vi "Error Query.vi"(8 "error in (no error)":errorcluster, 11 "VISA resource name":refnum<visa-resource-name>) -> (0 "error out":errorcluster, 1 "Error Message":string, 2 "Error":i32, 3 "VISA resource name out":refnum<visa-resource-name>)   [LabVIEW 2011, in "Agilent 4194.lvlib"]
doc: "This function reads an error code from the instrument's error queue.\n\nNotes:\n\n(1) For list of error messages see also operation manual.\n\n(2)This instrument does not return an error message string."
uses:
  <instrlib>/Agilent 4194/Agilent 4194.lvlib
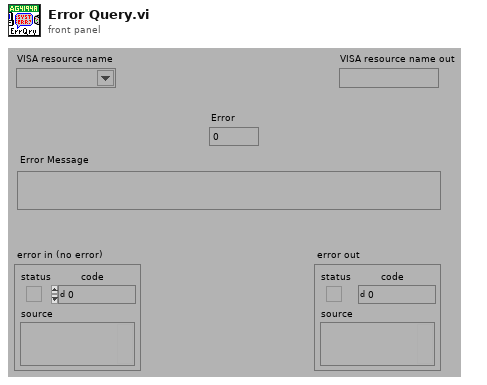
[diagram p1: front panel]
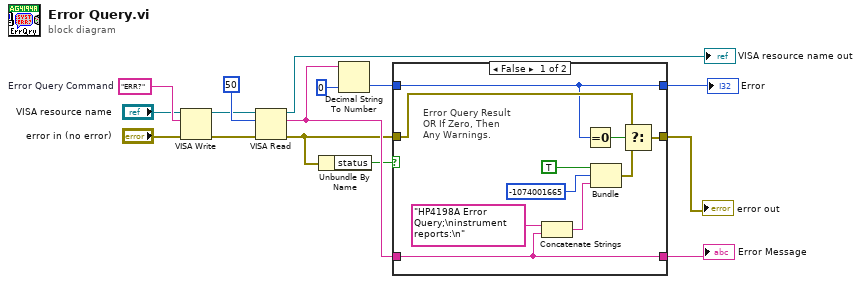
[diagram p0: block diagram]
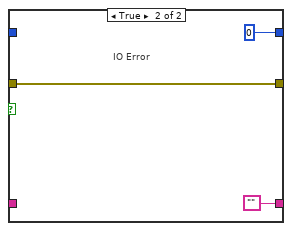
[diagram p2: hidden frame]
diagram:
  w11 = "ERR?"  # Error Query Command
  n1 = VISA Write(VISA resource name="VISA resource name", write buffer=w11, error in (no error)="error in (no error)") -> (VISA resource name out=w8:refnum<visa-resource-name>, error out=w10:errorcluster)  [unwired: 1 out]
  n2 = VISA Read(VISA resource name=w8, byte count=u32 50 ("Bytes"), error in (no error)=w10) -> (VISA resource name out=→"VISA resource name out":refnum<visa-resource-name>, read buffer=w13:string, error out=w7:errorcluster)  [unwired: 1 out]
  n3 = Unbundle By Name(w7) -> ("status"=w12:bool)
  n4 = Decimal String To Number(string=w13, default (0L)=0) -> (number=w15:i32)  [unwired: 1 in, 1 out]
  n5 = case shown="False" w12 {
    tunnel: w13 -> [w23 _]
    tunnel: w7 -> [w19 w28]
    tunnel: [w20 w28] -> w4
    tunnel: [w23 ""] -> w3
    tunnel: [w16 0] -> w2
    tunnel: w15 -> [w16 _]
    frame False {
      # "Error Query Result\nOR If Zero, Then\nAny Warnings."
      n6 = Concatenate Strings("HP4198A Error Query;\ninstrument reports:\n" ("Source"), w23) -> (w22:string)
      n7 = Equal To 0?(x=w16) -> (x = 0?=w17:bool)
      n8 = Bundle("Status"=TRUE, "Code"=-1074001665, w22) -> (w21:cluster{"Status":bool, "Code":i32, string})  [unwired: 1 in]
      n9 = Select(t=w19, s=w17, f=w21) -> (s? t:f=w20:errorcluster)
    }
    frame True {
      # "IO Error"
    }
  }
  "error out" <- w4
  "Error Message" <- w3
  "Error" <- w2
